vi "Test Render.vi"() -> ()   [LabVIEW 2010]
uses:
  <vilib>/Utility/miscctls.llb/LVRGBAColorTypeDef.ctl
  <vilib>/Utility/miscctls.llb/LV3DPointTypeDef.ctl
  <vilib>/picture/3D Picture Control/NI_3D Picture Control.lvlib
panel:
  in  "index":i32
  in  "Structures":T1(array[cluster])
  in  "Atom Size":dbl(slide) scale=0.0..1.0
  out "ModelView Matrix":sgl[][](array[numeric])
  out "Projection Matrix":sgl[][](array[numeric])
  out "Scene Display 2":refnum<vi>(3d-picture)
  in  "Target":T2 {"X" scale=0.0..10.0; "Y" scale=0.0..0.1; "Z" scale=0.0..10.0}
  in  "Scale":dbl(slide) scale=0.0..0.2
  in  "Camera Position":T2 {"X" scale=0.0..10.0; "Y" scale=0.0..10.0; "Z" scale=0.0..10.0}
  in  "Background Color":T3
  in  "Color":u32(colorbox)
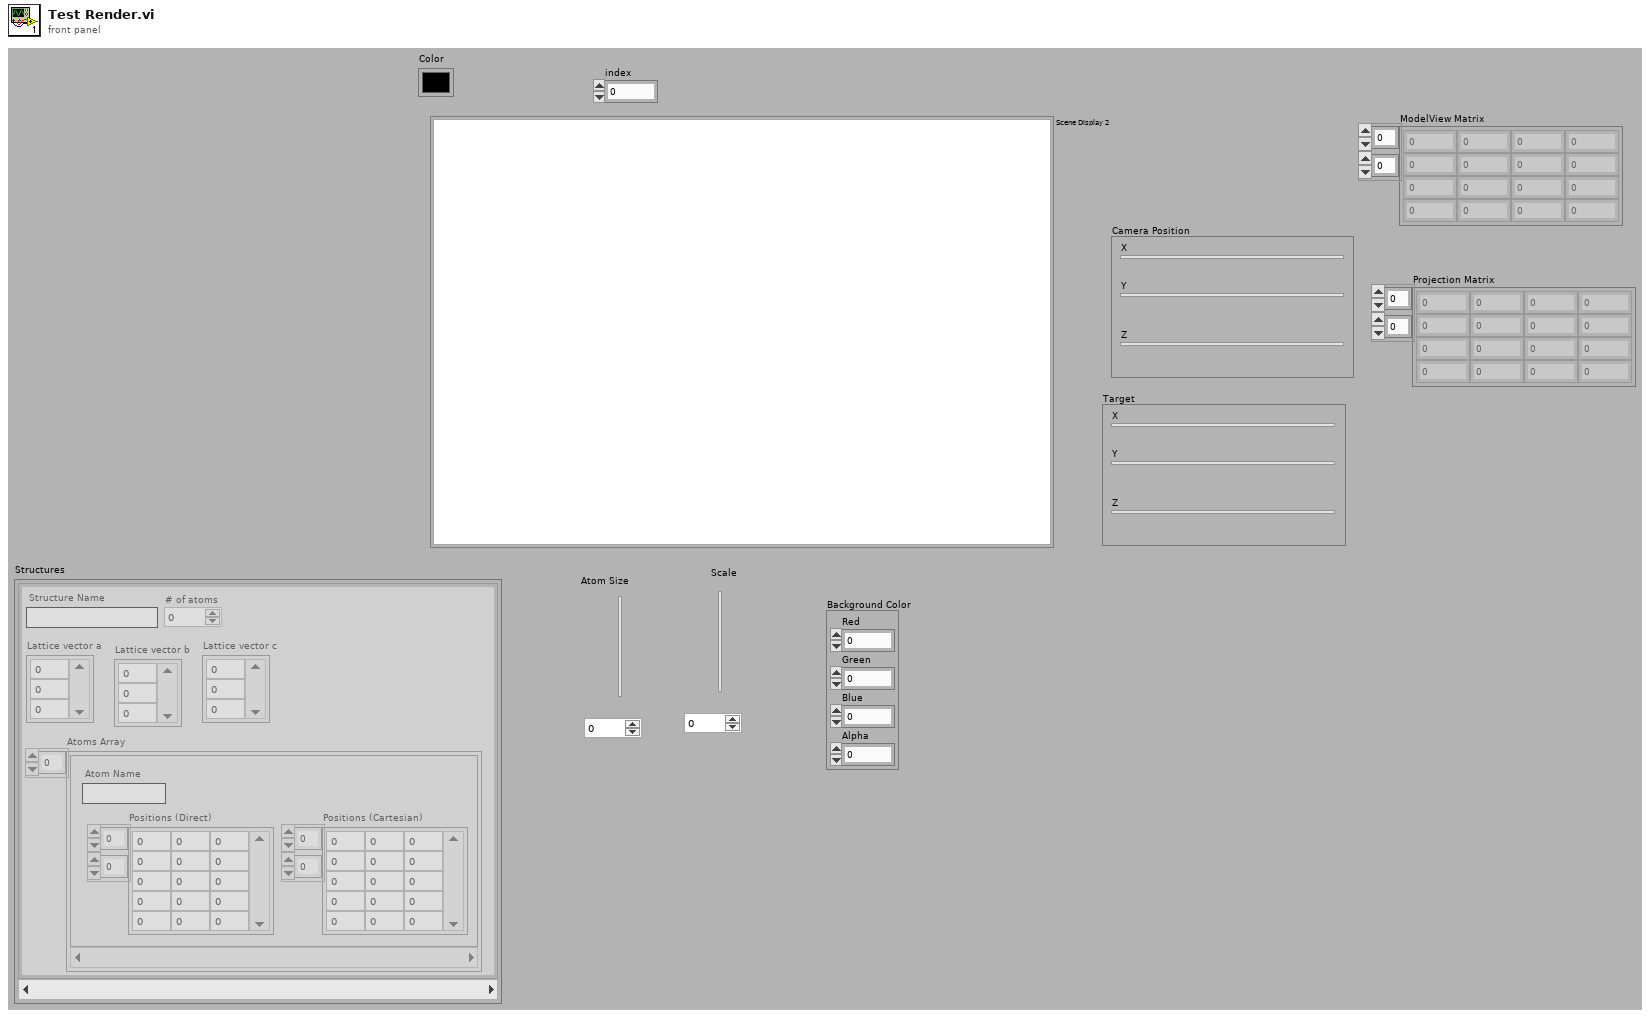
[diagram p1: front panel]
types:
  T1 = cluster{"Structure Name":string, "Lattice vector a":dbl[], "Lattice vector b":dbl[], "Lattice vector c":dbl[], "Atoms Array":cluster{"Atom Name":string, "Positions (Direct)":dbl[][], "Positions (Cartesian)":dbl[][]}[], "# of atoms":i32}[]
  T2 = typedef "LV3DPointTypeDef.ctl" = cluster{"X":sgl, "Y":sgl, "Z":sgl}
  T3 = typedef "LVRGBAColorTypeDef.ctl" = cluster{"Red":sgl, "Green":sgl, "Blue":sgl, "Alpha":sgl}
  T4 = cluster{"Red":sgl, "Green":sgl, "Blue":sgl, "Alpha":sgl}[]
  T5 = cluster{"Structure Name":string, "Lattice vector a":dbl[], "Lattice vector b":dbl[], "Lattice vector c":dbl[], "Atoms Array":cluster{"Atom Name":string, "Positions (Direct)":dbl[][], "Positions (Cartesian)":dbl[][]}[], "# of atoms":i32}
  T6 = cluster{"Atom Name":string, "Positions (Direct)":dbl[][], "Positions (Cartesian)":dbl[][]}[]
  T7 = cluster{"Positions (Cartesian)[0]":dbl, "Positions (Cartesian)[1]":dbl, "Positions (Cartesian)[2]":dbl}
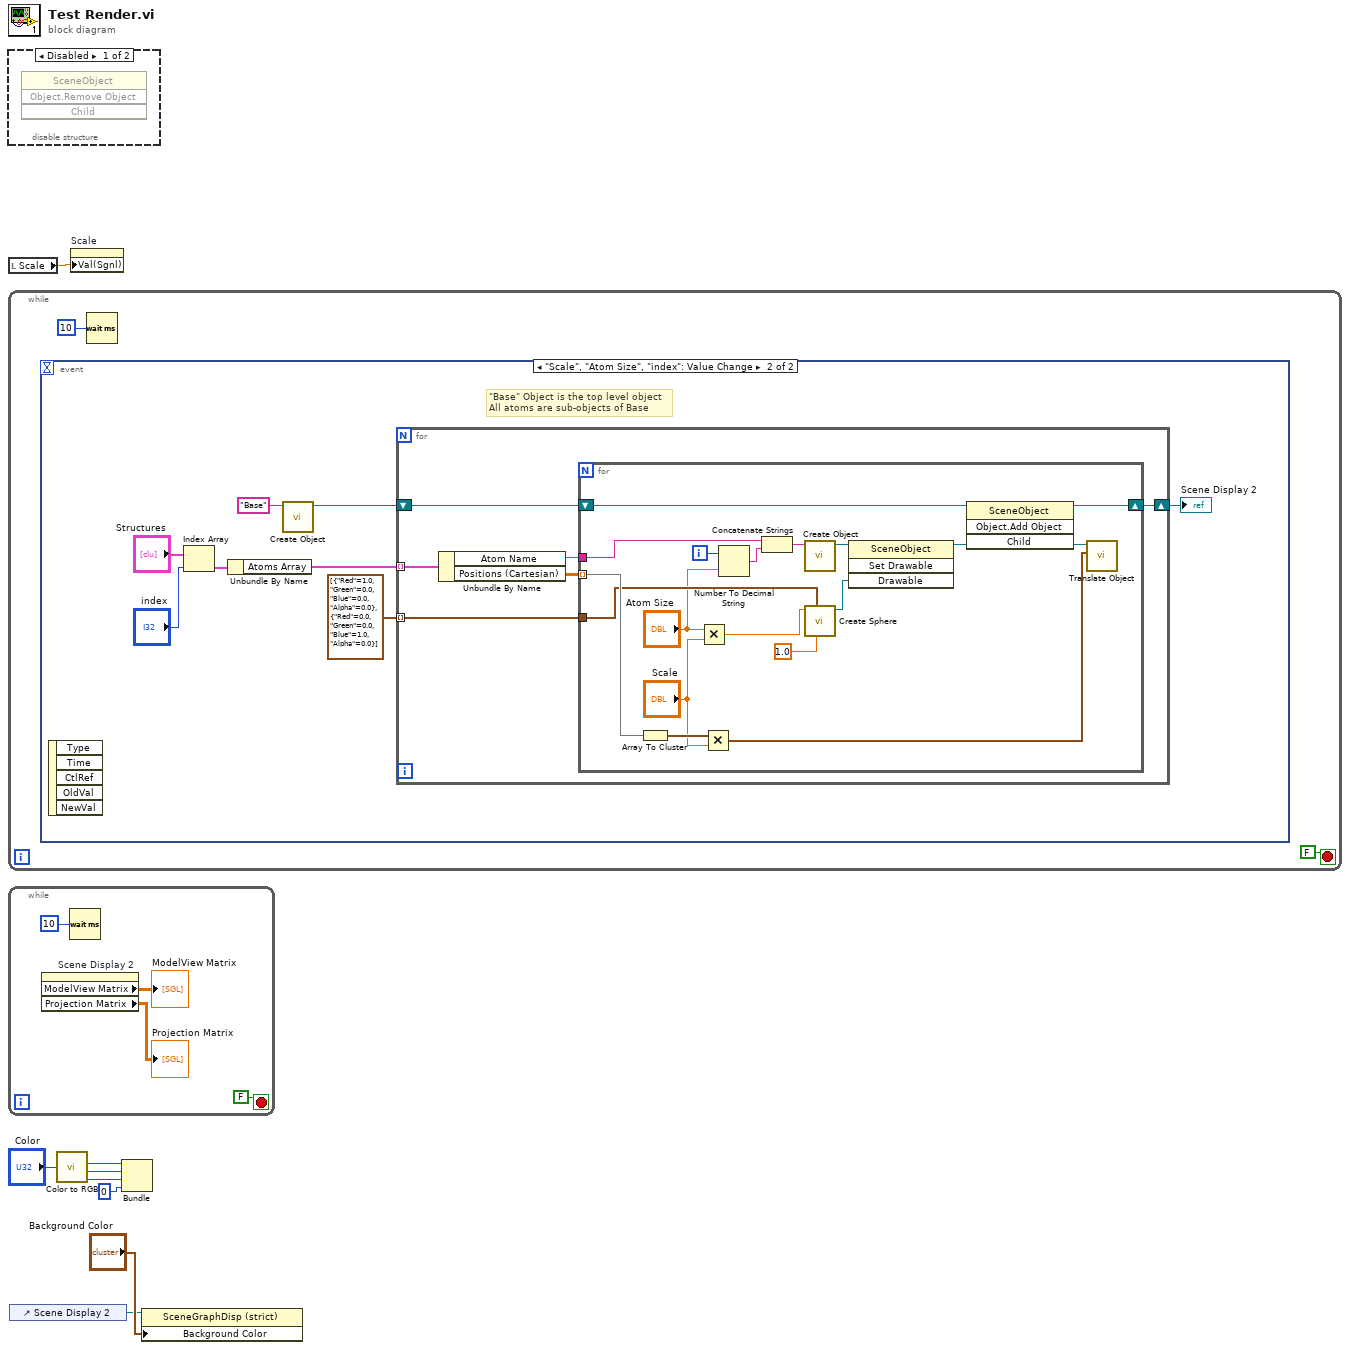
[diagram p0: block diagram]
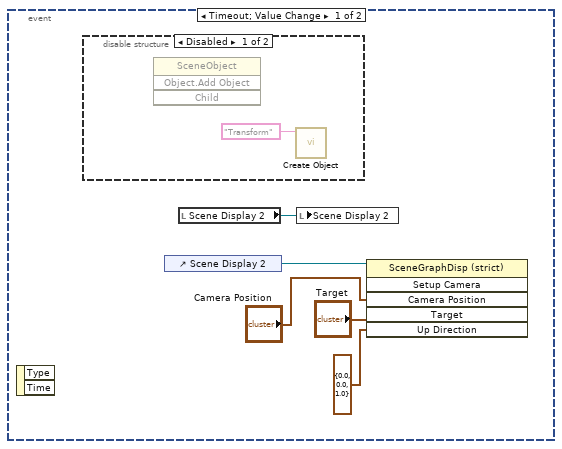
[diagram p3: hidden frame]
diagram:
  n1 = disable-structure shown="Disabled" {
    frame Disabled {
      n2 = invoke class="SceneObject" method="Object.Remove Object"() -> ()  [unwired: 4 in, 4 out]
    }
    frame Enabled {
    }
  }
  n3 = local read "Scale"() -> (w1:dbl)
  n4 = while {
    stop <- FALSE stop-if-true
    n5 = event shown="[1] \"Scale\", \"Atom Size\", \"index\": Value Change" {
      selector: _ -> [_ _]
      dyn-events: _ -> [_ _]
      timeout: _ -> [_ _]
      event Timeout; Value Change {
        n6 = event-data() -> ()  [unwired: 1 in, 2 out]
        n7 = disable-structure shown="Disabled" {
          frame Disabled {
            n8 = invoke class="SceneObject" method="Object.Add Object"() -> ()  [unwired: 4 in, 4 out]
            n9 = call <vilib>:"Create Object.vi"("Name"="Transform") -> ()  [unwired: 1 in, 10 out]
          }
          frame Enabled {
          }
        }
        n10 = control-ref of="Scene Display 2"() -> (w12:refnum<vi>)
        n11 = local read "Scene Display 2"() -> (w11:refnum<vi>)
        n12 = local write "Scene Display 2"(w11) -> ()
        n13 = invoke class="SceneGraphDisp (strict)" method="Setup Camera"(reference=w12, "Camera Position"="Camera Position", "Target"="Target", "Up Direction"=T2 {"X"=0.0, "Y"=0.0, "Z"=1.0}) -> ()  [unwired: 2 in, 6 out]
      }
      event "Scale", "Atom Size", "index": Value Change {
        # "\"Base\" Object is the top level object\nAll atoms are sub-objects of Base"
        n14 = event-data() -> ()  [unwired: 1 in, 5 out]
        n15 = Index Array(array="Structures", index="index") -> (element=w18:T5)
        n16 = Unbundle By Name(w18) -> ("Atoms Array"=w21:T6)
        n17 = call <vilib>:"Create Object.vi"("Name"="Base") -> ("Scene:New Object"=w24:refnum<vi>)  [unwired: 1 in, 9 out]
        n18 = for {
          tunnel: w21 -> [w30] mode=indexing
          shift-right: [w28] -> w20
          shift-left: w24 -> [w27]
          tunnel: T4 [{"Red"=1.0, "Green"=0.0, "Blue"=0.0, "Alpha"=0.0}, {"Red"=0.0, "Green"=0.0, "Blue"=1.0, "Alpha"=0.0}] -> [w25] mode=indexing
          n19 = Unbundle By Name(w30) -> ("Atom Name"=w29:string, "Positions (Cartesian)"=w26:dbl[][])
          n20 = for {
            tunnel: w29 -> [w46]
            tunnel: w26 -> [w39] mode=indexing
            shift-right: [w42] -> w28
            shift-left: w27 -> [w41]
            tunnel: w25 -> [w35]
            i -> [w38]
            n21 = Array To Cluster(array=w39) -> (cluster=w36:T7)
            n22 = Multiply(x="Atom Size", y="Scale") -> (x*y=w33:dbl)
            n23 = Multiply(x=w36, y="Scale") -> (x*y=w32:T7)
            n24 = Number To Decimal String(number=w38, width (-)="Atom Size") -> (decimal integer string=w47:string)
            n25 = Concatenate Strings(w46, w47) -> (w45:string)
            n26 = call <vilib>:"Create Object.vi"("Name"=w45) -> ("Scene:New Object"=w44:refnum<vi>)  [unwired: 1 in, 9 out]
            n27 = call <vilib>:"Create Sphere.vi"("Detail"=sgl 1.0, "Color"=w35, "Radius"=w33) -> ("New Sphere Refnum"=w43:refnum<vi>)  [unwired: 7 in, 1 out]
            n28 = invoke class="SceneObject" method="Set Drawable"(reference=w44, "Drawable"=w43) -> (reference out=w40:refnum<vi>)  [unwired: 2 in, 3 out]
            n29 = invoke class="SceneObject" method="Object.Add Object"(reference=w41, "Child"=w40) -> (reference out=w42:refnum<vi>, "Child"=w37:refnum<vi>)  [unwired: 2 in, 2 out]
            n30 = call <vilib>:"Translate Object.vi"("Translation"=w32, "Scene.Object In"=w37) -> ()  [unwired: 1 in, 9 out]
          }
        }
        "Scene Display 2" <- w20
      }
    }
    n31 = Wait (ms)(milliseconds to wait=u32 10) -> ()  [unwired: 1 out]
  }
  n32 = while {
    stop <- FALSE stop-if-true
    n33 = property on="Scene Display 2" class="SceneGraphDisp (strict)"() -> ("ModelView Matrix"=→"ModelView Matrix":sgl[][], "Projection Matrix"=→"Projection Matrix":sgl[][])  [unwired: 2 in, 2 out]
    n34 = Wait (ms)(milliseconds to wait=u32 10) -> ()  [unwired: 1 out]
  }
  n35 = control-ref of="Scene Display 2"() -> (w2:refnum<vi>)
  n36 = call <vilib>:"Color to RGB.vi"("Color"="Color") -> ("R"=w7:u8, "G"=w6:u8, "B"=w5:u8)  [unwired: 1 out]
  n37 = property on="Scale" class="Slide (strict)"("Val(Sgnl)"=w1) -> ()  [unwired: 2 in, 2 out]
  n38 = Bundle("R"=w7, "G"=w6, "B"=w5, "milliseconds to wait"=u32 0) -> ()  [unwired: 1 in, 1 out]
  n39 = property on="Property Node" class="SceneGraphDisp (strict)"(reference=w2, "Background Color"="Background Color") -> ()  [unwired: 1 in, 2 out]
